vi "TblCheck.vi"(4 "error in":errorcluster, 7 "connection reference":T1) -> (0 "error out":errorcluster, 2 "tables":string[](array[string]), 3 "conn ref out":T1)   [LabVIEW 2010]
uses:
  <vilib>/Addons/database/Connection.llb/Conn ObjectReference.ctl
  <vilib>/addons/database/Connection.llb/Conn Execute.vi
  <vilib>/addons/database/NI_Database_API.lvlib
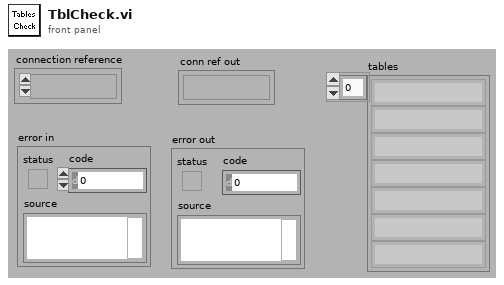
[diagram p1: front panel]
types:
  T1 = typedef "NI_Database_API.lvlib/Conn ObjectReference.ctl" = refnum<k1>
  T2 = cluster{"type":string, "units":string, "n":i32}[]
  T3 = typedef "NI_Database_API.lvlib/DB Tools Column Info.ctl" = cluster{"column name":string, "data type":T4, "size":i32, "allow null?":bool}
  T4 = typedef "NI_Database_API.lvlib/DB Tools DataTypes.ctl" = enum16{"String", "Long (I32)", "Single (SGL)", "Double (DBL)", "Date/Time", "Binary"}
  T5 = cluster{"key":string, "column information":T3[]}[]
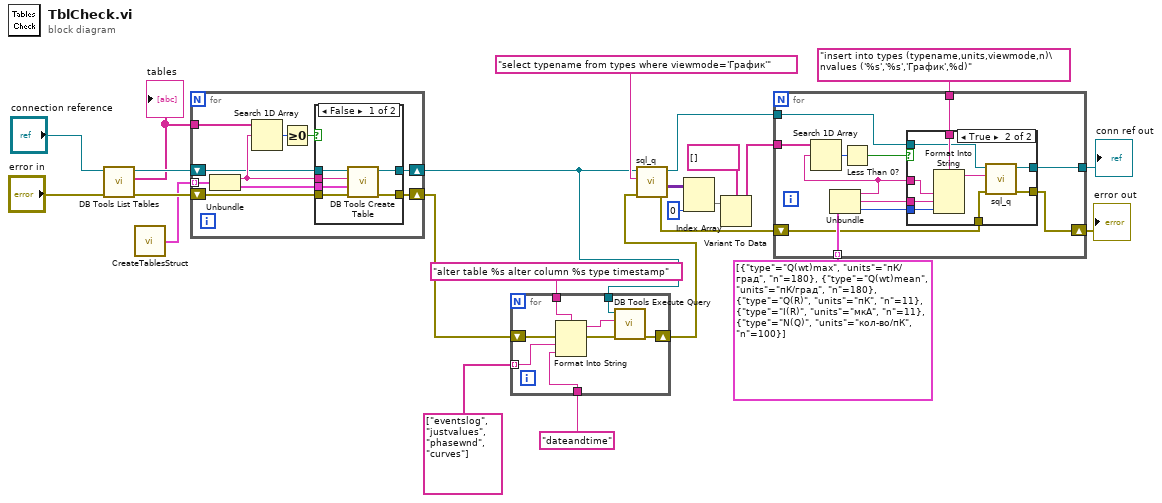
[diagram p0: block diagram]
diagram:
  n1 = call <vilib>:"DB Tools List Tables.vi"("error in (no error)"="error in", "connection reference"="connection reference") -> ("error out"=w23:errorcluster, "tables"=w22:string[], "connection reference out"=w24:T1)  [unwired: 3 in]
  "tables" <- w22
  n2 = call "CreateTablesStruct.vi"() -> ("Array"=w19:T5)
  n3 = for {
    tunnel: w19 -> [w31] mode=indexing
    tunnel: w22 -> [w34]
    shift-right: [w26] -> w5
    shift-left: w24 -> [w25]
    shift-right: [w28] -> w4
    shift-left: w23 -> [w27]
    n4 = Unbundle(w31) -> ("key"=w30:string, "column information"=w29:T3[])
    n5 = Search 1D Array(1D array=w34, element=w30) -> (index of element=w33:i32)  [unwired: 1 in]
    n6 = Greater Or Equal To 0?(x=w33) -> (x >= 0?=w32:bool)
    n7 = case shown="False" w32 {
      tunnel: w30 -> [w40 _]
      tunnel: w29 -> [w39 _]
      tunnel: [w38 w42] -> w28
      tunnel: w27 -> [w37 w42]
      tunnel: [w36 w41] -> w26
      tunnel: w25 -> [w35 w41]
      frame False {
        n8 = call <vilib>:"DB Tools Create Table.vi"("error in (no error)"=w37, "column information"=w39, "table"=w40, "connection reference"=w35) -> ("error out"=w38:errorcluster, "connection reference out"=w36:T1)  [unwired: 4 in]
      }
      frame True {
      }
    }
  }
  n9 = for {
    tunnel: "alter table %s alter column %s type timestamp" -> [w50]
    tunnel: w5 -> [w47]
    shift-right: [w46] -> w3
    shift-left: w4 -> [w45]
    tunnel: string[] ["eventslog", "justvalues", "phasewnd", "curves"] -> [w44] mode=indexing
    tunnel: "dateandtime" -> [w43]
    n10 = Format Into String(format string=w50, error in=w45, w44, w43) -> (resulting string=w48:string, error out=w49:errorcluster)  [unwired: 1 in]
    n11 = call-poly <vilib>:"DB Tools Execute Query.vi"("error in (no error)"=w49, "SQL query"=w48, "connection reference"=w47) -> ("error out"=w46:errorcluster)  [unwired: 5 in, 1 out]
  }
  n12 = call "sql_q.vi"("error in"=w3, "SQL query"="select typename from types where viewmode='График'", "connect ref"=w5) -> ("error out"=w9:errorcluster, "recordset data"=w15:variant[][], "conn ref out"=w10:T1)  [unwired: 1 in, 1 out]
  n13 = Index Array(array=w15, index (col)=0 ("disabled index (col)")) -> (element=w13:variant[])  [unwired: 1 in]
  n14 = Variant To Data(Variant=w13, type=string[] []) -> (data=w11:string[])  [unwired: 1 in, 1 out]
  n15 = for {
    tunnel: "insert into types (typename,units,viewmode,n)\nvalues ('%s','%s','График',%d)" -> [w62]
    tunnel: T2 [{"type"="Q(wt)max", "units"="пК/град", "n"=180}, {"type"="Q(wt)mean", "units"="пК/град", "n"=180}, {"type"="Q(R)", "units"="пК", "n"=11}, {"type"="I(R)", "units"="мкА", "n"=11}, {"type"="N(Q)", "units"="кол-во/пК", "n"=100}] -> [w59] mode=indexing
    tunnel: w11 -> [w61]
    tunnel: w10 -> [w54]
    shift-right: [w52] -> w7
    shift-left: w9 -> [w53]
    tunnel: [w51] -> w8
    n16 = Unbundle(w59) -> ("type"=w58:string, "units"=w57:string, "n"=w56:i32)
    n17 = Search 1D Array(1D array=w61, element=w58) -> (index of element=w60:i32)  [unwired: 1 in]
    n18 = Less Than 0?(x=w60) -> (x < 0?=w55:bool)
    n19 = case shown="True" w55 {
      tunnel: w62 -> [_ w73]
      tunnel: w58 -> [_ w71]
      tunnel: w57 -> [_ w70]
      tunnel: w56 -> [_ w69]
      tunnel: w54 -> [w63 w68]
      tunnel: w53 -> [w64 w67]
      tunnel: [w64 w66] -> w52
      tunnel: [w63 w65] -> w51
      frame False {
      }
      frame True {
        n20 = Format Into String(format string=w73, w71, w70, w69) -> (resulting string=w72:string)  [unwired: 2 in, 1 out]
        n21 = call "sql_q.vi"("error in"=w67, "SQL query"=w72, "connect ref"=w68) -> ("error out"=w66:errorcluster, "conn ref out"=w65:T1)  [unwired: 1 in, 2 out]
      }
    }
  }
  "error out" <- w7
  "conn ref out" <- w8
